vi "main.vi"(10 "Complex Number":T1) -> (1 "Phase (°)":dbl format="%#_4g", 2 "Magnitude":dbl)   [LabVIEW 2023]
doc: "Purpose:\nThis VI integrates the Magnitude VI and Phase VI to calculate and display both the magnitude and the phase of a complex number.\n\nInputs:\nComplex Number (complex): The input complex number, for which both the magnitude and phase will be calculated.\nOutputs:\nMagnitude (double): The absolute value (magnitude) of the complex number.\nPhase (double): The phase (argument) of the complex number in grad.\nFunctionality:\nThe VI takes a complex number as input.\nIt calls the Magnitude VI to calculate the magnitude.\nIt calls the Phase VI to compute the phase.\nBoth values (magnitude and phase) are displayed to the user on the front panel.\nExecution Notes:\nThis VI uses the results from both the Magnitude VI and Phase VI, so ensure that both subVIs are functioning correctly.\nResults are displayed in real-time as soon as the complex input is provided.\nThe phase is given in radians; you can convert it to degrees using additional processing if needed."
uses:
  controls/calculatePhaseControl.ctl
panel:
  in  "?":bool
  in  "?":bool
  # "OUTPUT VALUES"
  # "INPUT VALUE"
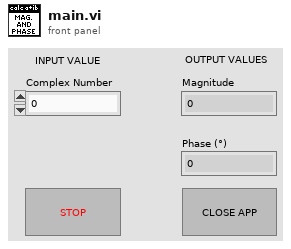
[diagram p1: front panel]
types:
  T1 = typedef "calculatePhaseControl.ctl" = csg
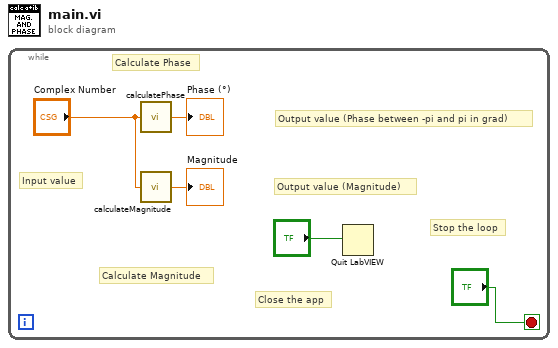
[diagram p0: block diagram]
diagram:
  n1 = while {
    stop <- "?" stop-if-true
    # "Close the app"
    # "Stop the loop"
    # "Output value (Magnitude)"
    # "Output value (Phase between -pi and pi in grad)"
    # "Input value"
    # "Calculate Magnitude"
    # "Calculate Phase"
    n2 = call "calculatePhase.vi"("input"="Complex Number") -> ("output"=→"Phase (°)":dbl)
    n3 = call "calculateMagnitude.vi"("input"="Complex Number") -> ("output"=→"Magnitude":dbl)
    n4 = Quit LabVIEW(quit? (T)="?") -> ()
  }
